vi "Parse Labels and Com Arrays.vi"(5 "All Confgured Com Array":u8[](array[numeric])=[100, 2, 3, 4, 5, 6, 7, 8, 9, 10, 11, 12, 13, 14, 15, 16, 17, 18, 19, 20, 21, 22, 23, 24, 25, 26, 27, 28, 29, 30, 31, 32, 33, 34, 35, 36, 37, 38, 39, 40, 41, 42, 43, 44, 45, 46, 47, 48, 49, 50, 51, 52, 53, 54, 55, 56], 7 "Station Labels":string[](array[string])) -> (1 "Labels1":string[](array[string]), 2 "Com1":u8[](array[numeric]), 3 "Labels1A":string[](array[string]), 4 "Com1a":u8[](array[numeric]), 6 "Labels2":string[](array[string]), 8 "Com2":u8[](array[numeric]), 10 "Labels3":string[](array[string]), 13 "Com4":u8[](array[numeric]), 14 "Labels4":string[](array[string]), 15 "Com3":u8[](array[numeric]))   [LabVIEW 2012]
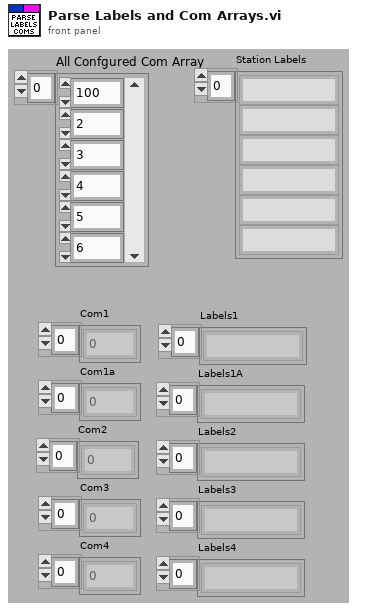
[diagram p1: front panel]
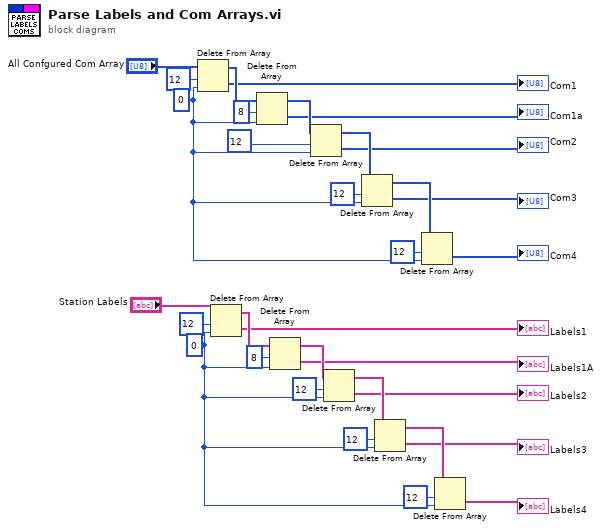
[diagram p0: block diagram]
diagram:
  w2 = 0 ("index")
  w1 = 0 ("index")
  n1 = Delete From Array(array="All Confgured Com Array", length=12, index=w1) -> (deleted portion=→"Com1":u8[], array with subset deleted=w30:u8[])
  n2 = Delete From Array(array="Station Labels", length=12, index=w2) -> (deleted portion=→"Labels1":string[], array with subset deleted=w16:string[])
  n3 = Delete From Array(array=w30, length=8, index=w1) -> (deleted portion=→"Com1a":u8[], array with subset deleted=w26:u8[])
  n4 = Delete From Array(array=w16, length=8, index=w2) -> (deleted portion=→"Labels1A":string[], array with subset deleted=w19:string[])
  n5 = Delete From Array(array=w26, length=12, index=w1) -> (deleted portion=→"Com2":u8[], array with subset deleted=w25:u8[])
  n6 = Delete From Array(array=w19, length=12, index=w2) -> (deleted portion=→"Labels2":string[], array with subset deleted=w20:string[])
  n7 = Delete From Array(array=w25, length=12, index=w1) -> (deleted portion=→"Com3":u8[], array with subset deleted=w24:u8[])
  n8 = Delete From Array(array=w20, length=12, index=w2) -> (deleted portion=→"Labels3":string[], array with subset deleted=w21:string[])
  n9 = Delete From Array(array=w24, length=12, index=w1) -> (deleted portion=→"Com4":u8[])  [unwired: 1 out]
  n10 = Delete From Array(array=w21, length=12, index=w2) -> (deleted portion=→"Labels4":string[])  [unwired: 1 out]
